vi "MU Write Switch Command.vi"(8 "error in (no error)":errorcluster, 9 "rplNew":u32, 10 "modeaNew":u32, 11 "handle":u64) -> (0 "error out (no error)":errorcluster, 3 "function return":u32)   [LabVIEW 2017, in "MU_3SL_interface.lvlib"]
uses:
  MU_3SL_interface.lvlib
  lib/MU_3SL_interface.dll
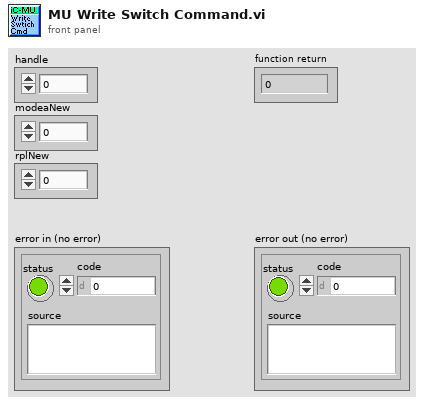
[diagram p1: front panel]
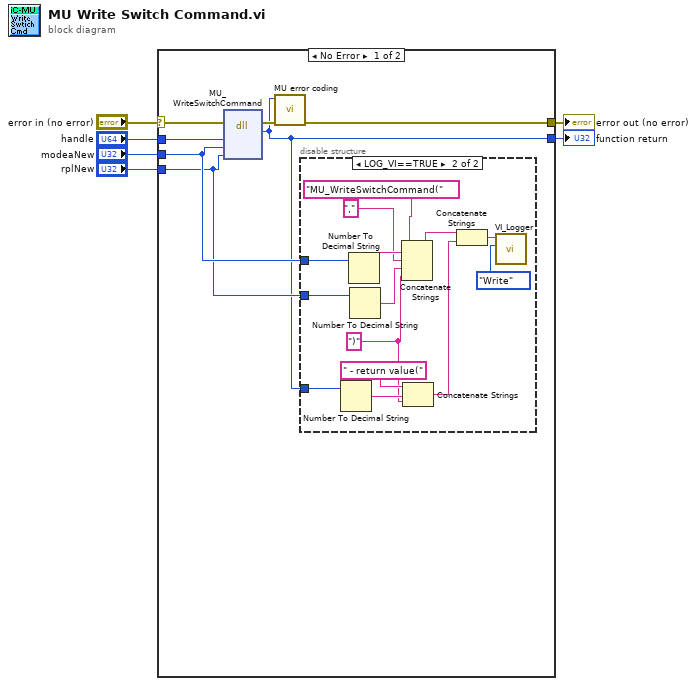
[diagram p0: block diagram]
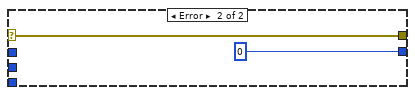
[diagram p3: hidden frame]
diagram:
  n1 = case shown="No Error" "error in (no error)" {
    selector: "error in (no error)" -> [w10 w29]
    tunnel: [w7 u32 0] -> w6
    tunnel: "handle" -> [w13 _]
    tunnel: "modeaNew" -> [w9 _]
    tunnel: "rplNew" -> [w8 _]
    tunnel: [w11 w29] -> w2
    frame No Error {
      n2 = dll-call lib="C:/Users/bes/AppData/Roaming/work/mu_9so/icsubmodules/soft_mu_3sl_master/lv_interface/lib/MU_3SL_interface**.*" fn="MU_WriteSwitchCommand"(error in=w10, "handle"=w13, "modeaNew"=w9, "rplNew"=w8) -> (error out=w12:errorcluster, "return type"=w7:u32)  [unwired: 5 in, 1 out]
      n3 = call "MU error coding.vi"("error in (no error)"=w12, "function return in"=w7) -> ("error out"=w11:errorcluster)  [unwired: 9 in]
      n4 = disable-structure shown="LOG_VI==TRUE" {
        disable-tunnel: w7 -> [_ w25]
        disable-tunnel: w9 -> [_ w20]
        disable-tunnel: w8 -> [_ w17]
        frame condition #0 {
        }
        frame condition #1 (active) {
          w14 = ")" ("string")
          n5 = Number To Decimal String(number=w25) -> (decimal integer string=w24:string)  [unwired: 1 in]
          n6 = Number To Decimal String(number=w20) -> (decimal integer string=w19:string)  [unwired: 1 in]
          n7 = Number To Decimal String(number=w17) -> (decimal integer string=w16:string)  [unwired: 1 in]
          n8 = Concatenate Strings("MU_WriteSwitchCommand(" ("Info in"), w19, "," ("string"), w16, w14) -> (w23:string)
          n9 = Concatenate Strings(" - return value(" ("string"), w24, w14) -> (w22:string)
          n10 = Concatenate Strings(w23, w22) -> (w21:string)
          n11 = call "VI_Logger.vi"("Action (Read)"=enum16{"Write", "Read"}."Write", "Info in"=w21) -> ()  [unwired: 8 in, 2 out]
        }
      }
    }
    frame Error {
    }
  }
  "function return" <- w6
  "error out (no error)" <- w2
